vi "Download.vi"(7 "Node-ID":u8, 8 "error in":errorcluster, 9 "Data":u8[](array[numeric]) format="%02x", 10 "Multiplexer":cluster{"Index":u16, "Sub-Index":u8} {"Index" format="%.0x"}, 11 "Service Data Object in":refnum<class "Service Data Object.lvclass">) -> (0 "error out":errorcluster, 1 "Request":refnum<class "CANopen Request Message.lvclass">, 2 "Expected Response":refnum<class "CANopen Response Message.lvclass">, 3 "Service Data Object out":refnum<class "Service Data Object.lvclass">)   [LabVIEW 2024, in "Service Data Object.lvclass"]
uses:
  Service Data Object.lvclass
  Service Data Object.lvclass/Service Data Object.ctl
  Initiate Down-Upload Response Comparator/Initiate Down-Upload Response Comparator.lvclass
  <vilib>/Utility/Data Type/NI_Data Type.lvlib
  SDO Response Compare Strategy/SDO Response Compare Strategy.lvclass
  CANopen Response/CANopen Response Message.lvclass
  CANopen Request/CANopen Request Message.lvclass
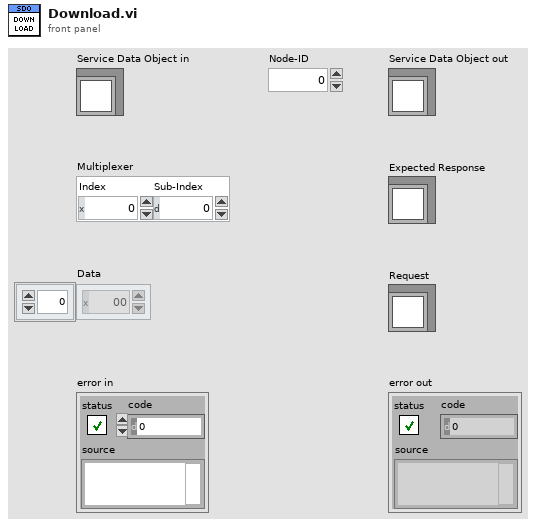
[diagram p1: front panel]
types:
  T1 = typedef "NI_Data Type.lvlib/Data Type.ctl" = enum8{"Invalid Type", "Void", "I8", "I16", "I32", "I64", "U8", "U16", "U32", "U64", "Single Float", "Double Float", "Extended Float", "Single Complex", "Double Complex", "Extended Complex", "Enum U8", "Enum U16", "Enum U32", "Enum U64", "Single Float With Unit", "Double Float With Unit", "Extended Float With Unit", "Single Complex with Unit", "Double Complex with Unit", "Extended Complex with Unit", "Boolean", "String", "Path", "Picture", "Tag", "Array", "Cluster", "Variant", "LV Variant", "Waveform", "Timestamp", "Digital Waveform", "Digital Data", "ExpressData", "Refnum", "External Data", "VI", "Poly VI", "LabVIEW Class Instance", "Fixed Point", "Set Collection", "Map Collection"}
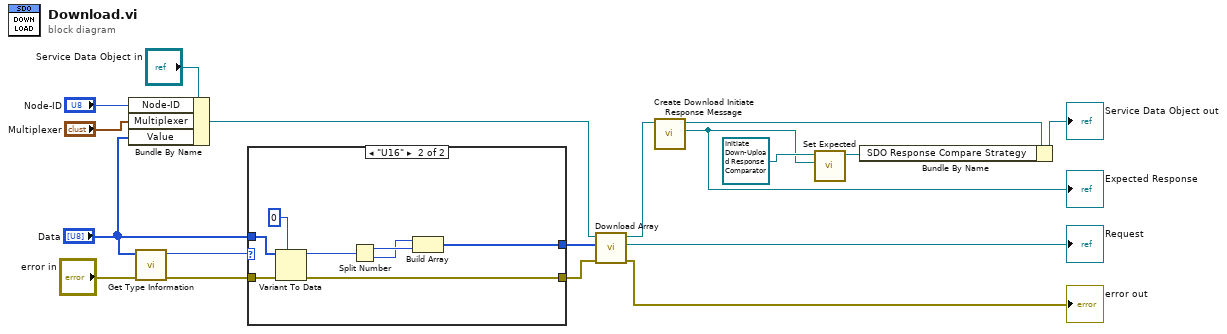
[diagram p0: block diagram]
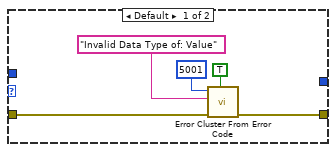
[diagram p2: hidden frame]
diagram:
  n1 = Bundle By Name(cluster="Service Data Object in", "Node-ID"="Node-ID", "Multiplexer"="Multiplexer", "Value"="Data") -> (w15:refnum<class "Service Data Object.lvclass">)
  n2 = call <vilib>:"Get Type Information.vi"("error in (no error)"="error in", "variant"="Data") -> ("error out"=w14:errorcluster, "type"=w18:T1)  [unwired: 5 in, 3 out]
  n3 = case shown="\"U16\"" w18 {
    tunnel: "Data" -> [_ w31]
    tunnel: w14 -> [w23 w30]
    tunnel: [w19 w25] -> w5
    tunnel: [_ w24] -> w4
    frame Default {
      n4 = call <vilib>:"Error Cluster From Error Code.vi"("show call chain? (False)"=TRUE, "error in (no error)"=w23, "error message (\"\")"="Invalid Data Type of: Value" ("error message (\"\")"), "error code (0)"=5001) -> ("error out"=w19:errorcluster)  [unwired: 5 in]
    }
    frame "U16" {
      n5 = Variant To Data(error in=w30, type=u16 0, Variant=w31) -> (data=w26:u16, error out=w25:errorcluster)
      n6 = Split Number(x=w26) -> (hi(x)=w28:u8, lo(x)=w27:u8)
      n7 = Build Array(w27, w28) -> (w24:u8[])
    }
  }
  n8 = call "Download Array.vi"("error in"=w5, "Data"=w4, "Service Data Object in"=w15) -> ("error out"=→"error out":errorcluster, "CANopen Message out"=→"Request":refnum<class "CANopen Request Message.lvclass">, "Service Data Object out"=w1:refnum<class "Service Data Object.lvclass">)  [unwired: 6 in]
  n9 = call "Create Download Initiate Response Message.vi"("Service Data Object in"=w1) -> ("CANopen Response Message"=w7:refnum<class "CANopen Response Message.lvclass">, "Service Data Object out"=w6:refnum<class "Service Data Object.lvclass">)  [unwired: 9 in]
  "Expected Response" <- w7
  n10 = call "Set Expected.vi"("CANopen Message"=w7, "SDO Response Compare Strategy in"=refnum<class "Initiate Down-Upload Response Comparator.lvclass"> refnum ("CANopen Master.lvlib:Initiate Down-Upload Response Comparator.lvclass")) -> ("SDO Response Compare Strategy out"=w8:refnum<class "Initiate Down-Upload Response Comparator.lvclass">)  [unwired: 9 in]
  n11 = Bundle By Name(cluster=w6, "SDO Response Compare Strategy"=w8) -> (→"Service Data Object out":refnum<class "Service Data Object.lvclass">)
